vi "S1500_S7Com_OPEN(SubVI).vi"(0 "remote address":string, 1 "remote port":u16=102, 2 "timeout ms":i32=500, 3 "error in (no error)":errorcluster) -> (4 "Connection Confirm CC":T1 format="X%02x", 5 "connection ID out":refnum<k5>, 6 "PDU Response":T1 format="X%02x", 7 "Error":bool, 8 "error out":errorcluster)   [LabVIEW 2018]
doc: "Opens an S7 Connection with a PLC."
uses:
  S1500_test_S7Com_HexByteArray.ctl
  S1500_S7Com_HexByte.ctl
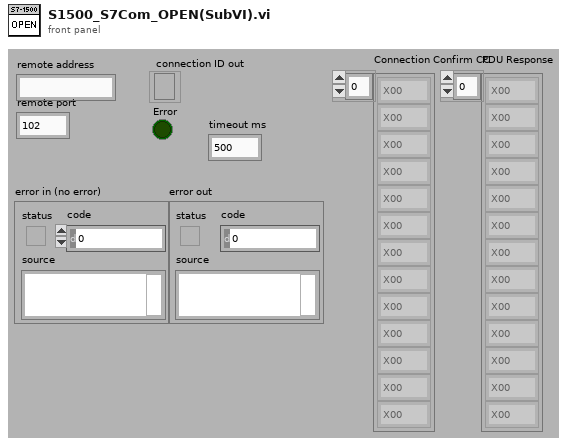
[diagram p1: front panel]
types:
  T1 = typedef "S1500_test_S7Com_HexByteArray.ctl" = T2[]
  T2 = typedef "S1500_S7Com_HexByte.ctl" = u8
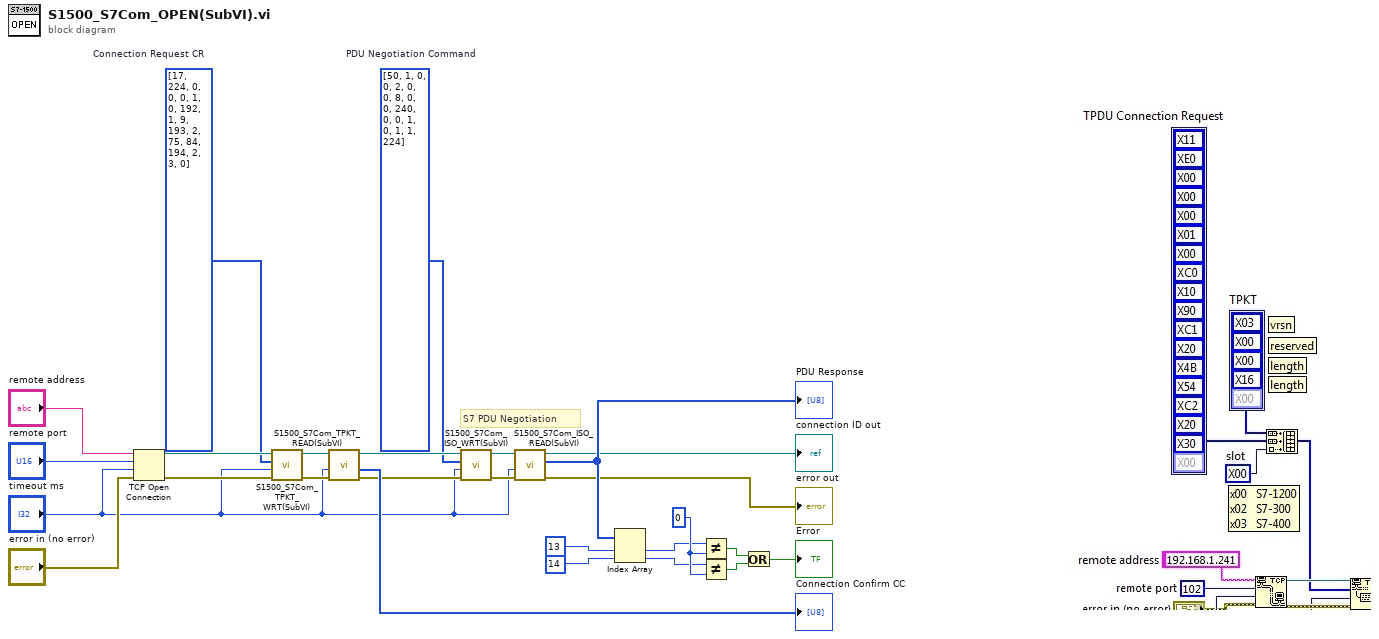
[diagram p0: block diagram]
diagram:
  w1 = T1 [17, 224, 0, 0, 0, 1, 0, 192, 1, 9, 193, 2, 75, 84, 194, 2, 3, 0]  # Connection Request CR
  w3 = T1 [50, 1, 0, 0, 2, 0, 0, 8, 0, 0, 240, 0, 0, 1, 0, 1, 1, 224]  # PDU Negotiation Command
  w25 = u8 0
  # "S7 PDU Negotiation"
  n1 = TCP Open Connection(address="remote address", remote port or service name="remote port", timeout ms (60000)="timeout ms", error in (no error)="error in (no error)") -> (connection ID=w15:refnum<k5>, error out=w6:errorcluster)  [unwired: 1 out]
  n2 = call "S1500_S7Com_TPKT_WRT(SubVI).vi"("error in"=w6, "timeout ms"="timeout ms", "TPDU_In"=w1, "connection ID in"=w15) -> ("error out"=w14:errorcluster, "connection ID out"=w13:refnum<k5>)  [unwired: 2 out]
  n3 = call "S1500_S7Com_TPKT_READ(SubVI).vi"("error in"=w14, "timeout ms (25000)"="timeout ms", "connection ID in"=w13) -> ("error out"=w5:errorcluster, "TPDU Data"=→"Connection Confirm CC":T1, "connection ID out"=w16:refnum<k5>)  [unwired: 2 out]
  n4 = call "S1500_S7Com_ISO_WRT(SubVI).vi"("error in"=w5, "timeout ms (25000)"="timeout ms", "TPDU_In"=w3, "connection ID in"=w16) -> ("error out"=w11:errorcluster, "connection ID out"=w12:refnum<k5>)  [unwired: 2 out]
  n5 = call "S1500_S7Com_ISO_READ(SubVI).vi"("error in"=w11, "timeout ms (25000)"="timeout ms", "connection ID in"=w12) -> ("error out"=→"error out":errorcluster, "TPDU Data"=w18:T1, "connection ID out"=→"connection ID out":refnum<k5>)  [unwired: 2 out]
  "PDU Response" <- w18
  n6 = Index Array(array=w18, index #1=13, index #2=14) -> (element #1=w23:T2, element #2=w24:T2)
  n7 = Not Equal?(x=w23, y=w25) -> (x != y?=w21:bool)
  n8 = Not Equal?(x=w24, y=w25) -> (x != y?=w22:bool)
  n9 = Or(x=w21, y=w22) -> (x .or. y?=→"Error":bool)
